vi "Read_Chan_Value_Gen.vi"(10 "Desired Ch Names":string[](array[string]), 11 "Raw data file":path) -> (2 "Values":string[](array[string]))   [LabVIEW 2011]
uses:
  Globals/Meas_global.vi
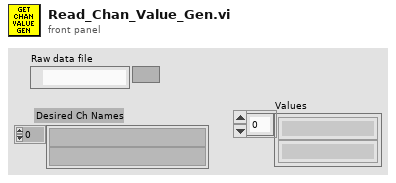
[diagram p1: front panel]
types:
  T1 = typedef "Post_Process.ctl" = enum16{"Take New Data", "Post Process Raw Data File"}
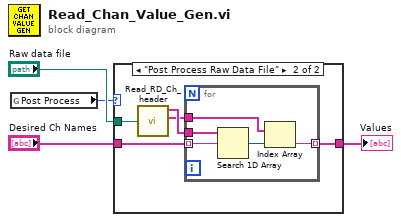
[diagram p0: block diagram]
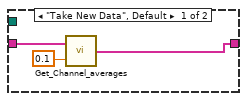
[diagram p2: hidden frame]
diagram:
  n1 = global read "Meas_global.vi" "Post Process"() -> (w3:T1)
  n2 = case shown="\"Post Process Raw Data File\"" w3 {
    tunnel: "Raw data file" -> [_ w12]
    tunnel: [w6 w8] -> w2
    tunnel: "Desired Ch Names" -> [w5 w9]
    frame "Take New Data", Default {
      n3 = call "Get_Channel_averages.vi"("Desired Ch Names"=w5, "Averaging time (mins)"=0.1) -> ("Values"=w6:string[])  [unwired: 1 in, 2 out]
    }
    frame "Post Process Raw Data File" {
      n4 = call "Read_RD_Ch_header.vi"("Raw data file"=w12) -> ("Ch Name Out"=w11:string[], "Ch Values"=w10:string[])  [unwired: 2 out]
      n5 = for {
        tunnel: w11 -> [w17]
        tunnel: w10 -> [w16]
        tunnel: w9 -> [w14] mode=indexing
        tunnel: [w13] -> w8 mode=indexing
        n6 = Search 1D Array(1D array=w17, element=w14) -> (index of element=w15:i32)  [unwired: 1 in]
        n7 = Index Array(array=w16, index=w15) -> (element=w13:string)
      }
    }
  }
  "Values" <- w2
